vi "Write Steering Frame.vi"(6 "Teleop command":T1, 8 "error in (no error)":errorcluster, 11 "ROV in":refnum<class "ROV Host.lvclass">) -> (0 "error out":errorcluster, 3 "ROV out":refnum<class "ROV Host.lvclass">)   [LabVIEW 2012, in "ROV Host.lvclass"]
uses:
  ROV Host.lvclass
  Support/Teleop command.ctl
  ROV Host.lvclass/ROV Host.ctl
  <vilib>/robotics/Steering/Steering Frame/NI_Robotics_Steering Frame.lvclass/NI_Robotics_Steering Frame.ctl
  <vilib>/robotics/Steering/Steering Frame/Get Steering Frame Velocity from Wheels.vi
  <vilib>/robotics/Steering/Steering Frame/NI_Robotics_Steering Frame.lvclass
  <vilib>/robotics/Steering/Steering Frame/Get Steering Frame Velocity from Motors.vi
  <vilib>/robotics/Steering/Steering Frame/Apply Steering Frame Velocity to Wheels.vi
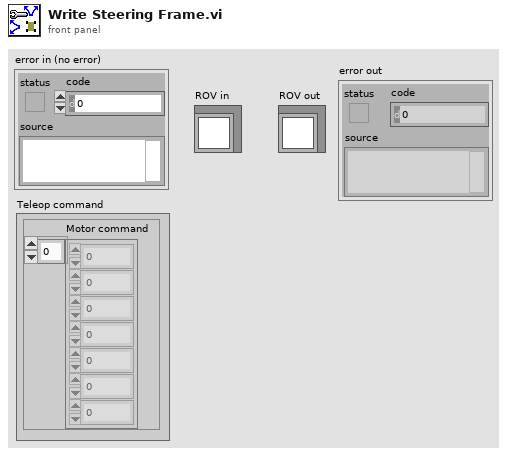
[diagram p1: front panel]
types:
  T1 = typedef "Teleop command.ctl" = cluster{"Motor command":dbl[]}
  T2 = typedef "NI_Robotics_Steering Class Types.lvlib/Mecanum Steering Frame.ctl" = refnum<class "NI_Robotics_Mecanum Steering Frame.lvclass">
  T3 = typedef "NI_Robotics_Steering Class Types.lvlib/Differential Steering Frame.ctl" = refnum<class "NI_Robotics_Differential Steering Frame.lvclass">
  T4 = typedef "NI_Robotics_Wheel.lvclass/Wheel State.ctl" = cluster{"wheel name":string, "forward angular velocity":dbl, "caster angular velocity":dbl, "caster wheel angle (rad)":dbl, "steering angle (rad)":dbl}
  T5 = cluster{"mecanum steering frame out":T2, "differential steering frame out":T3}
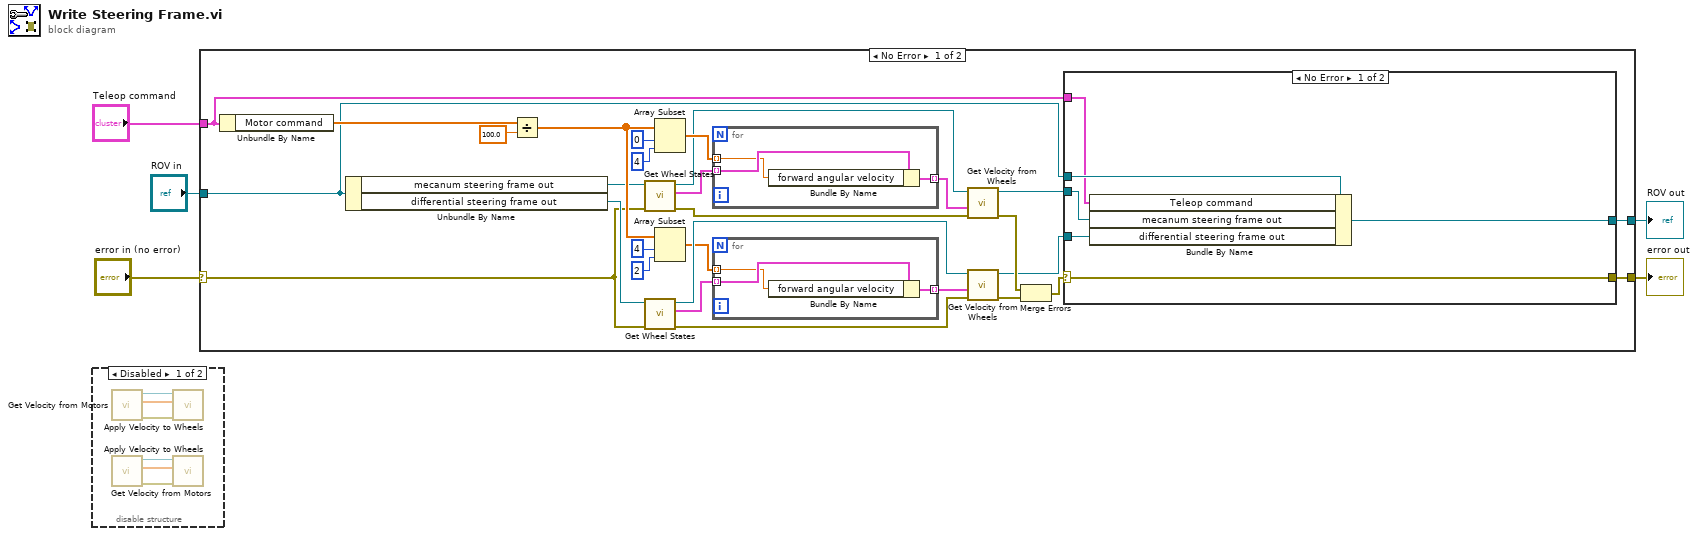
[diagram p0: block diagram]
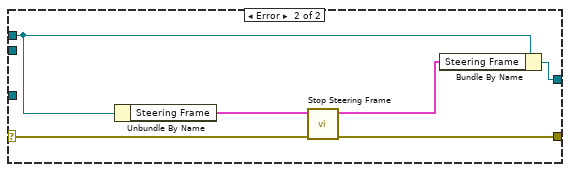
[diagram p3: hidden frame]
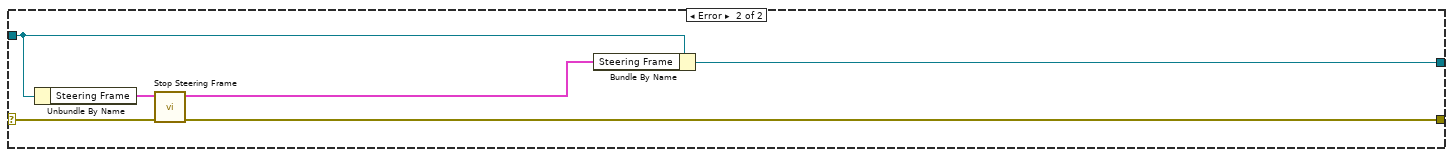
[diagram p4: hidden frame]
diagram:
  n1 = disable-structure shown="Disabled" {
    frame Disabled {
      n2 = call-poly <vilib>:"Get Velocity from Motors.vi"() -> ("error out"=w8:errorcluster, "estimated steering frame velocity"=w6:dbl[], "steering frame out"=w7:refnum<class "NI_Robotics_Steering Frame.lvclass">)  [unwired: 9 in]
      n3 = call-poly <vilib>:"Get Velocity from Motors.vi"() -> ("error out"=w9:errorcluster, "estimated steering frame velocity"=w10:dbl[], "steering frame out"=w11:refnum<class "NI_Robotics_Steering Frame.lvclass">)  [unwired: 9 in]
      n4 = call-poly <vilib>:"Apply Velocity to Wheels.vi"("error in (no error)"=w8, "steering frame velocity"=w6, "steering frame in"=w7) -> ("error out"=w12:errorcluster)  [unwired: 5 in, 3 out]
      n5 = call-poly <vilib>:"Apply Velocity to Wheels.vi"("error in (no error)"=w9, "steering frame velocity"=w10, "steering frame in"=w11) -> ("error out"=w13:errorcluster)  [unwired: 5 in, 3 out]
    }
    frame Enabled {
    }
  }
  n6 = case shown="No Error" "error in (no error)" {
    selector: "error in (no error)" -> [w17 w66]
    tunnel: [w32 w65] -> w4
    tunnel: "Teleop command" -> [w34 _]
    tunnel: "ROV in" -> [w33 w62]
    tunnel: [w31 w61] -> w1
    frame No Error {
      n7 = Unbundle By Name(w34) -> ("Motor command"=w37:dbl[])
      n8 = Unbundle By Name(w33) -> ("mecanum steering frame out"=w30:T2, "differential steering frame out"=w18:T3)
      n9 = Divide(x=w37, y=100.0) -> (x/y=w36:dbl[])
      n10 = call <vilib>:"Get Wheel States.vi"("error in (no error)"=w17, "steering frame in"=w30) -> ("error out"=w26:errorcluster, "wheel states"=w29:T4[], "steering frame out"=w25:T2)  [unwired: 7 in]
      n11 = call <vilib>:"Get Wheel States.vi"("error in (no error)"=w17, "steering frame in"=w18) -> ("error out"=w15:errorcluster, "wheel states"=w21:T4[], "steering frame out"=w20:T3)  [unwired: 7 in]
      n12 = Array Subset(array=w36, index=0, length=4) -> (w28:dbl[])
      n13 = Array Subset(array=w36, index=4, length=2) -> (w14:dbl[])
      n14 = for {
        tunnel: w29 -> [w48] mode=indexing
        tunnel: w28 -> [w47] mode=indexing
        tunnel: [w46] -> w27 mode=indexing
        n15 = Bundle By Name(cluster=w48, "forward angular velocity"=w47) -> (w46:T4)
      }
      n16 = for {
        tunnel: w21 -> [w45] mode=indexing
        tunnel: w14 -> [w44] mode=indexing
        tunnel: [w43] -> w22 mode=indexing
        n17 = Bundle By Name(cluster=w45, "forward angular velocity"=w44) -> (w43:T4)
      }
      n18 = call-poly <vilib>:"Get Velocity from Wheels.vi"("error in (no error)"=w26, "acquired wheel states"=w27, "steering frame in"=w25) -> ("error out"=w23:errorcluster, "steering frame out"=w24:T2)  [unwired: 5 in, 2 out]
      n19 = call-poly <vilib>:"Get Velocity from Wheels.vi"("error in (no error)"=w15, "acquired wheel states"=w22, "steering frame in"=w20) -> ("error out"=w16:errorcluster, "steering frame out"=w19:T3)  [unwired: 5 in, 2 out]
      n20 = Merge Errors(w23, w16) -> (w35:errorcluster)
      n21 = case shown="No Error" w35 {
        selector: w35 -> [w52 w57]
        tunnel: w34 -> [w51 _]
        tunnel: w33 -> [w54 w58]
        tunnel: [w52 w56] -> w32
        tunnel: [w53 w55] -> w31
        tunnel: w24 -> [w50 _]
        tunnel: w19 -> [w49 _]
        frame No Error {
          n22 = Bundle By Name(cluster=w54, "Teleop command"=w51, "mecanum steering frame out"=w50, "differential steering frame out"=w49) -> (w53:refnum<class "ROV Host.lvclass">)
        }
        frame Error {
          n23 = Unbundle By Name(w58) -> ("Steering Frame"=w59:T5)
          n24 = call "Stop Steering Frame.vi"("error in (no error)"=w57, "Steering Frame in"=w59) -> ("error out"=w56:errorcluster, "Steering Frame out"=w60:T5)  [unwired: 8 in]
          n25 = Bundle By Name(cluster=w58, "Steering Frame"=w60) -> (w55:refnum<class "ROV Host.lvclass">)
        }
      }
    }
    frame Error {
      n26 = Unbundle By Name(w62) -> ("Steering Frame"=w63:T5)
      n27 = call "Stop Steering Frame.vi"("error in (no error)"=w66, "Steering Frame in"=w63) -> ("error out"=w65:errorcluster, "Steering Frame out"=w64:T5)  [unwired: 8 in]
      n28 = Bundle By Name(cluster=w62, "Steering Frame"=w64) -> (w61:refnum<class "ROV Host.lvclass">)
    }
  }
  "error out" <- w4
  "ROV out" <- w1
